vi "Broadcast Message.vi"(8 "error in (no error)":errorcluster, 9 "Message Data":variant, 10 "Message":string, 11 "Process In":refnum<class "Debug Process.lvclass">) -> (0 "error out":errorcluster, 3 "Process Out":refnum<class "Debug Process.lvclass">)   [LabVIEW 2020, in "Debug Process.lvclass"]
doc: "Send a broadcast message to any observer who has registered for broadcast messages."
uses:
  Debug Process.lvclass
  Broadcast Message Cluster.ctl
  Debug Process.lvclass/Debug Process.ctl
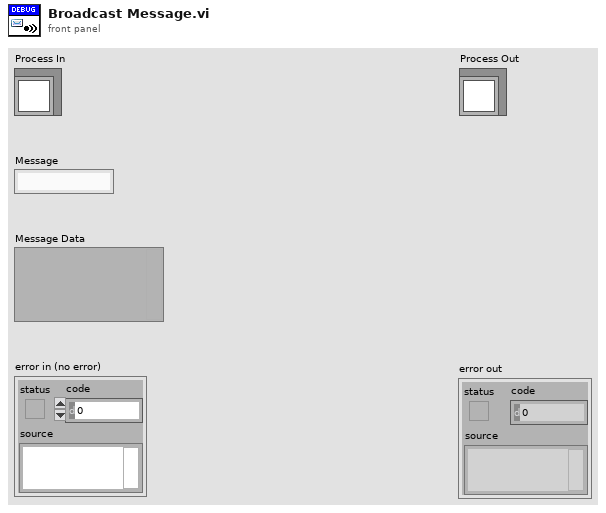
[diagram p1: front panel]
types:
  T1 = typedef "Debug Process.lvclass/Broadcast Message Cluster.ctl" = cluster{"Sender":string, "Message":string, "Message Data":variant}
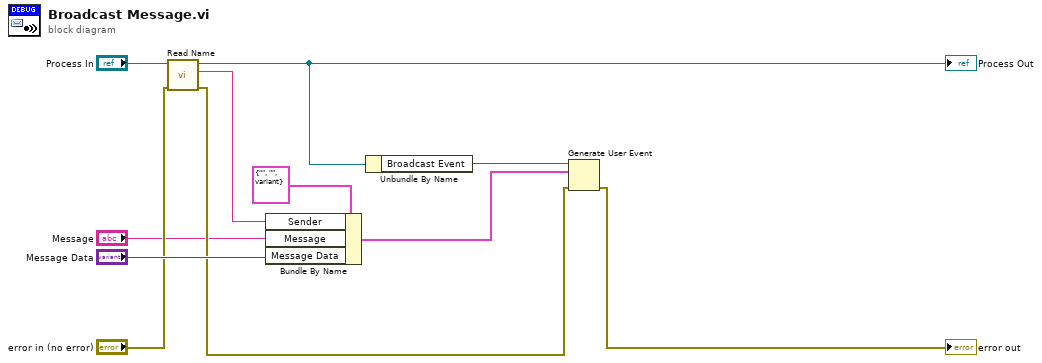
[diagram p0: block diagram]
diagram:
  n1 = call "Read Name.vi"("error in (no error)"="error in (no error)", "Process In"="Process In") -> ("error out"=w2:errorcluster, "Name"=w4:string, "Process Out"=w5:refnum<class "Debug Process.lvclass">)  [unwired: 7 in]
  "Process Out" <- w5
  n2 = Bundle By Name(cluster=T1 {"Sender"="", "Message"="", "Message Data"=variant} ("event data"), "Sender"=w4, "Message"="Message", "Message Data"="Message Data") -> (w7:T1)
  n3 = Unbundle By Name(w5) -> ("Broadcast Event"=w10:refnum<user-event>)
  n4 = Generate User Event(user event=w10, event data cluster=w7, error in=w2) -> (error out=→"error out":errorcluster)  [unwired: 1 in, 1 out]
